vi "test Parse Timestamp Array.vi"(11 "Test Case In":refnum<class "Test Named Fields Parser.lvclass">) -> (0 "error out":errorcluster, 3 "Test Case Out":refnum<class "Test Named Fields Parser.lvclass">)   [LabVIEW 2024, in "Test Named Fields Parser.lvclass"]
uses:
  Test Named Fields Parser.lvclass
  Test Named Fields Parser.lvclass/Test Named Fields Parser.ctl
  4993e8ee-a06a-463a-9684-69129f64d5ce.vi
  CSV Parser/Named Fields Parser/Named Fields Parser.lvclass
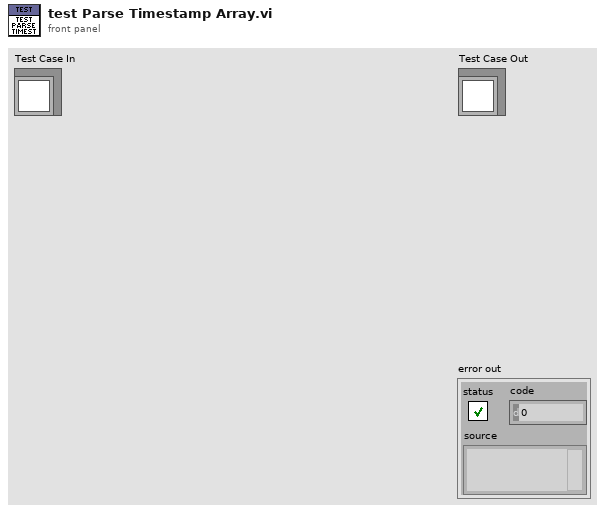
[diagram p1: front panel]
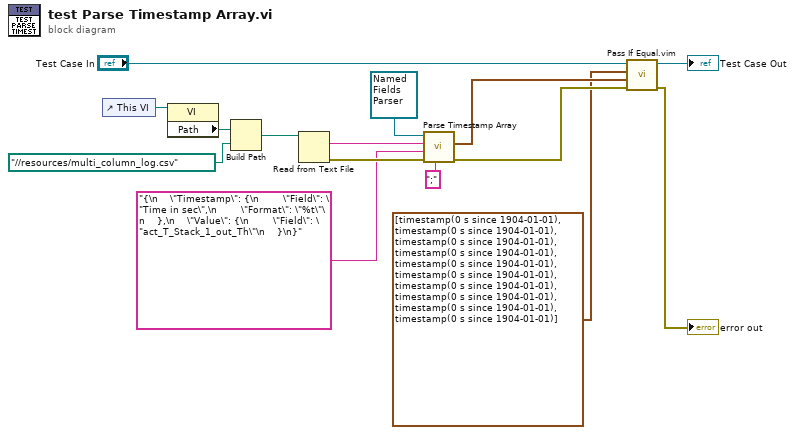
[diagram p0: block diagram]
diagram:
  n1 = control-ref of="This VI"() -> (w12:refnum<vi>)
  n2 = property class="VI"(reference=w12) -> ("Path"=w11:path)  [unwired: 1 in, 2 out]
  n3 = Build Path(base path=w11, name or relative path=path "../../resources/multi_column_log.csv" ("file (use dialog)")) -> (appended path=w10:path)
  n4 = Read from Text File(file (use dialog)=w10) -> (text=w9:string, error out=w8:errorcluster)  [unwired: 3 in, 2 out]
  n5 = call-dynamic "Parse Timestamp Array.vi"("Seperator"=";", "error in"=w8, "Input"="{\n    \"Timestamp\": {\n        \"Field\": \"Time in sec\",\n        \"Format\": \"%t\"\n    },\n    \"Value\": {\n        \"Field\": \"act_T_Stack_1_out_Th\"\n    }\n}" ("Input <JSON>"), "csv string"=w9, "Named Columns Parser in"=refnum<class "Named Fields Parser.lvclass"> refnum) -> ("error out"=w5:errorcluster, "Timestamp Array"=w3:timestamp[])  [unwired: 4 in, 1 out]
  n6 = call "Pass If Equal.vim"("error in (no error)"=w5, "Actual"=w3, "Expected"=timestamp[] [timestamp(0 s since 1904-01-01), timestamp(0 s since 1904-01-01), timestamp(0.099836 s since 1904-01-01), timestamp(0.201114 s since 1904-01-01), timestamp(0.300982 s since 1904-01-01), timestamp(0.400523 s since 1904-01-01), timestamp(0.500431 s since 1904-01-01), timestamp(0.601341 s since 1904-01-01), timestamp(0.700389 s since 1904-01-01), timestamp(0.801359 s since 1904-01-01)] ("Timestamp Array"), "LUnit Test Case In"="Test Case In") -> ("error out"=→"error out":errorcluster, "LUnit Test Case Out"=→"Test Case Out":refnum<class "Test Named Fields Parser.lvclass">)  [unwired: 6 in]
